vi "Update Line Final State.vi"(8 "error in (no error)":errorcluster, 9 "Output Line":i32, 10 "Final State":enum16{"Default", "High", "Low", "Same"}(ring), 11 "Master Device in":refnum<class "Master Device.lvclass">) -> (0 "error out":errorcluster, 3 "Master Device out":refnum<class "Master Device.lvclass">)   [LabVIEW 2013, in "Master Device.lvclass"]
uses:
  Master Device.lvclass
  Master Device.lvclass/Master Device.ctl
  <vilib>/Utility/error.llb/DialogType.ctl
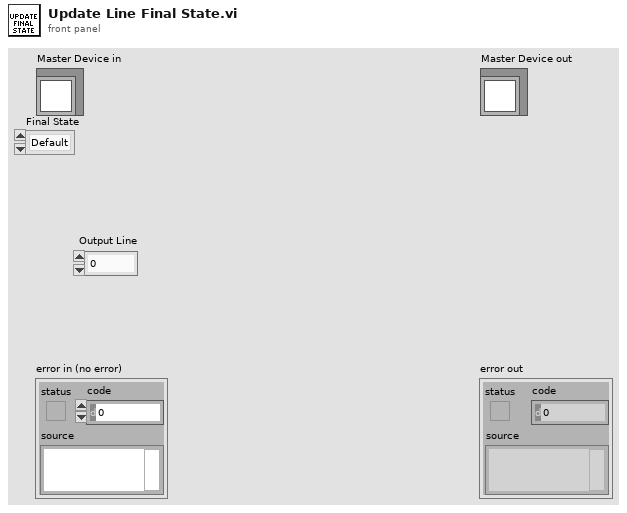
[diagram p1: front panel]
types:
  T1 = typedef "DialogType.ctl" = u16
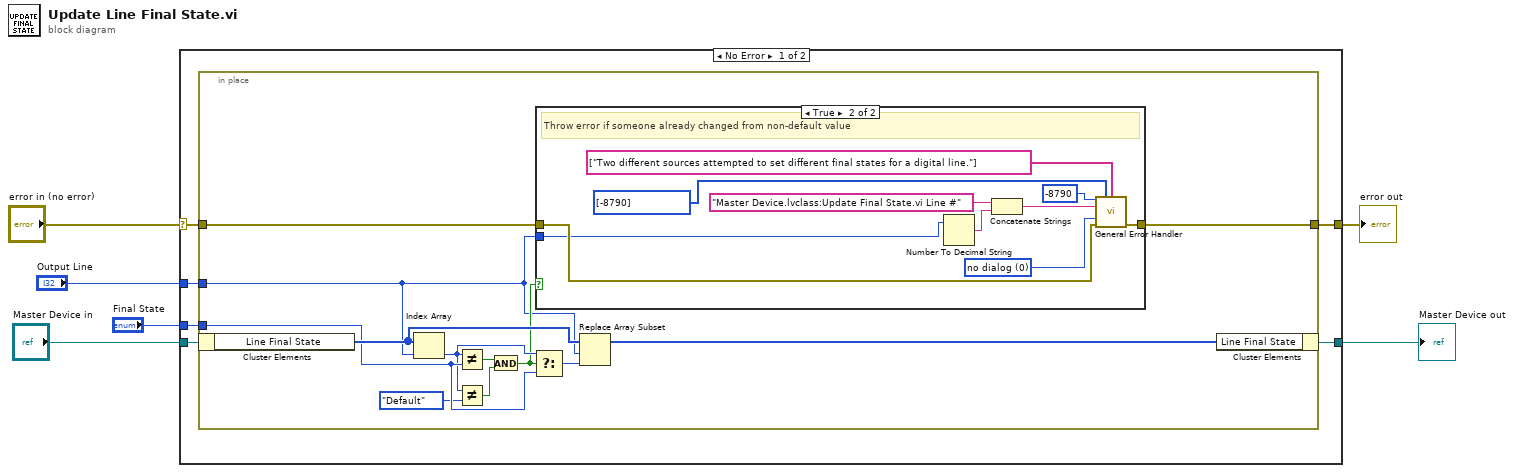
[diagram p0: block diagram]
diagram:
  n1 = case shown="No Error" "error in (no error)" {
    selector: "error in (no error)" -> [w8 w36]
    tunnel: [w7 w36] -> w5
    tunnel: [w11 w37] -> w3
    tunnel: "Master Device in" -> [w12 w37]
    tunnel: "Output Line" -> [w10 _]
    tunnel: "Final State" -> [w9 _]
    frame No Error {
      n2 = in-place {
        in-place-border: w10 -> [w13]
        in-place-border: w9 -> [w21]
        in-place-border: w8 -> [w16]
        in-place-border: [w14] -> w7
        # "Throw error if someone already changed from non-default value"
        n3 = in-place-cluster #1(w12) -> ("Line Final State"=w24:enum16{"Default", "High", "Low", "Same"}[])
        n4 = Index Array(array=w24, index=w13) -> (element=w20:enum16{"Default", "High", "Low", "Same"})
        n5 = Not Equal?(x=w20, y=w21) -> (x != y?=w18:bool)
        n6 = Not Equal?(x=w20, y=enum16{"Default", "High", "Low", "Same"}."Default" ("Final State")) -> (x != y?=w17:bool)
        n7 = And(x=w18, y=w17) -> (x .and. y?=w15:bool)
        n8 = Select(t=w20, s=w15, f=w21) -> (s? t:f=w22:enum16{"Default", "High", "Low", "Same"})
        n9 = case shown="True" w15 {
          tunnel: w16 -> [w25 w34]
          tunnel: [w25 w35] -> w14
          tunnel: w13 -> [_ w27]
          frame False {
            # "No problem, value was changed"
          }
          frame True {
            w33 = T1 0 items=["no dialog", "OK message", "continue or stop message", "OK message + warnings", "continue/stop + warnings"] ("type of dialog (OK msg:1)")
            # "Throw error if someone already changed from non-default value"
            n10 = Number To Decimal String(number=w27) -> (decimal integer string=w26:string)  [unwired: 1 in]
            n11 = Concatenate Strings("Master Device.lvclass:Update Final State.vi Line #" ("[error source] (\" \")"), w26) -> (w28:string)
            n12 = call <vilib>:"General Error Handler.vi"("[error code] (0)"=-8790, "[user-defined codes]"=i32[] [-8790], "[user-defined descriptions]"=string[] ["Two different sources attempted to set different final states for a digital line."], "[error source] (\" \")"=w28, "type of dialog (OK msg:1)"=w33, "error in (no error)"=w34) -> ("error out"=w35:errorcluster)  [unwired: 5 in, 4 out]
          }
        }
        n13 = Replace Array Subset(array=w24, new element=w22, index=w13) -> (w23:enum16{"Default", "High", "Low", "Same"}[])
        n14 = in-place-cluster #1("Line Final State"=w23) -> (w11:refnum<class "Master Device.lvclass">)
      }
    }
    frame Error {
    }
  }
  "error out" <- w5
  "Master Device out" <- w3
